vi "DDS_Check_Box.vi"(8 "error in (no error)":errorcluster, 10 "box #":i32, 11 "DDS Settings":T1={"Enable DDS"=TRUE, "Array of DDS Boxes"=[{"DDS box device reference"={"NI USB-8451 device reference"="USB0::0x3923::0x7166::01574F57::RAW", "DIO port"=0, "Serial Clock Rate [kHz]"=1000}, "Array of DDS Channels (4)"=[{"Power"=TRUE, "Channel Parameters"={"Ref Clock Rate [kHz]"=1000.0, "Full Scale Output\nPower [dBm]"=0.0}, "RAM Enable"=FALSE, "RAM Dest Type"=0, "RAM Default"={"Frequency [MHz]"="20", "Amplitude [dBm]"="-15", "Phase Offset [rad]"="0"}, "Array of DDS Profiles (8)"=[{"Single Tone"={"Frequency [MHz]"="75", "Amplitude [dBm]"="0", "Phase Offset [rad]"="0"}, "RAM Mode "=enum."Ramp Up", "Zero-crossing"=FALSE, "No Dwell High"=FALSE, "Function/Static"=TRUE, "RAM Function Settings"=["10*x", "1", "1", "260", "10"], "RAM Static Array"=[0.0], "Description"=""}, {"Single Tone"={"Frequency [MHz]"="200", "Amplitude [dBm]"="0", "Phase Offset [rad]"="0"}, "RAM Mode "=enum."Direct Switch", "Zero-crossing"=FALSE, "No Dwell High"=FALSE, "Function/Static"=FALSE, "RAM Function Settings"=["", "", "", "", "1"], "RAM Static Array"=[0.0], "Description"=""}, {"Single Tone"={"Frequency [MHz]"="", "Amplitude [dBm]"="", "Phase Offset [rad]"="0"}, "RAM Mode "=enum."Direct Switch", "Zero-crossing"=FALSE, "No Dwell High"=FALSE, "Function/Static"=FALSE, "RAM Function Settings"=["", "", "", "", "1"], "RAM Static Array"=[0.0], "Description"=""}, {"Single Tone"={"Frequency [MHz]"="", "Amplitude [dBm]"="0", "Phase Offset [rad]"="0"}, "RAM Mode "=enum."Ramp Up", "Zero-crossing"=FALSE, "No Dwell High"=FALSE, "Function/Static"=FALSE, "RAM Function Settings"=["10*x", "1", "1", "260", "10"], "RAM Static Array"=[0.0], "Description"=""}, {"Single Tone"={"Frequency [MHz]"="0", "Amplitude [dBm]"="-50", "Phase Offset [rad]"="0"}, "RAM Mode "=enum."Direct Switch", "Zero-crossing"=FALSE, "No Dwell High"=FALSE, "Function/Static"=FALSE, "RAM Function Settings"=["", "", "", "", "1"], "RAM Static Array"=[0.0], "Description"=""}, {"Single Tone"={"Frequency [MHz]"="0", "Amplitude [dBm]"="-50", "Phase Offset [rad]"="0"}, "RAM Mode "=enum."Direct Switch", "Zero-crossing"=FALSE, "No Dwell High"=FALSE, "Function/Static"=FALSE, "RAM Function Settings"=["", "", "", "", "1"], "RAM Static Array"=[0.0], "Description"=""}, {"Single Tone"={"Frequency [MHz]"="0", "Amplitude [dBm]"="-50", "Phase Offset [rad]"="0"}, "RAM Mode "=enum."Direct Switch", "Zero-crossing"=FALSE, "No Dwell High"=FALSE, "Function/Static"=FALSE, "RAM Function Settings"=["", "", "", "", "1"], "RAM Static Array"=[0.0], "Description"=""}, {"Single Tone"={"Frequency [MHz]"="0", "Amplitude [dBm]"="-50", "Phase Offset [rad]"="0"}, "RAM Mode "=enum."Direct Switch", "Zero-crossing"=FALSE, "No Dwell High"=FALSE, "Function/Static"=FALSE, "RAM Function Settings"=["", "", "", "", "1"], "RAM Static Array"=[0.0], "Description"=""}], "Description"=""}, {"Power"=TRUE, "Channel Parameters"={"Ref Clock Rate [kHz]"=1000.0, "Full Scale Output\nPower [dBm]"=0.0}, "RAM Enable"=FALSE, "RAM Dest Type"=0, "RAM Default"={"Frequency [MHz]"="", "Amplitude [dBm]"="-50", "Phase Offset [rad]"=""}, "Array of DDS Profiles (8)"=[{"Single Tone"={"Frequency [MHz]"="278.5", "Amplitude [dBm]"="0", "Phase Offset [rad]"="0"}, "RAM Mode "=enum."Direct Switch", "Zero-crossing"=FALSE, "No Dwell High"=FALSE, "Function/Static"=TRUE, "RAM Function Settings"=["", "", "", "", "1"], "RAM Static Array"=[0.0], "Description"=""}, {"Single Tone"={"Frequency [MHz]"="278.5", "Amplitude [dBm]"="-150", "Phase Offset [rad]"="0"}, "RAM Mode "=enum."Direct Switch", "Zero-crossing"=FALSE, "No Dwell High"=FALSE, "Function/Static"=FALSE, "RAM Function Settings"=["", "", "", "", "1"], "RAM Static Array"=[0.0], "Description"=""}, {"Single Tone"={"Frequency [MHz]"="278.5", "Amplitude [dBm]"="-10", "Phase Offset [rad]"="0"}, "RAM Mode "=enum."Direct Switch", "Zero-crossing"=FALSE, "No Dwell High"=FALSE, "Function/Static"=FALSE, "RAM Function Settings"=["", "", "", "", "1"], "RAM Static Array"=[0.0], "Description"=""}, {"Single Tone"={"Frequency [MHz]"="278.5", "Amplitude [dBm]"="-10", "Phase Offset [rad]"="0"}, "RAM Mode "=enum."Direct Switch", "Zero-crossing"=FALSE, "No Dwell High"=FALSE, "Function/Static"=FALSE, "RAM Function Settings"=["", "", "", "", "1"], "RAM Static Array"=[0.0], "Description"=""}, {"Single Tone"={"Frequency [MHz]"="60", "Amplitude [dBm]"="-50", "Phase Offset [rad]"="0"}, "RAM Mode "=enum."Direct Switch", "Zero-crossing"=FALSE, "No Dwell High"=FALSE, "Function/Static"=FALSE, "RAM Function Settings"=["", "", "", "", "1"], "RAM Static Array"=[0.0], "Description"=""}, {"Single Tone"={"Frequency [MHz]"="70", "Amplitude [dBm]"="-50", "Phase Offset [rad]"="0"}, "RAM Mode "=enum."Direct Switch", "Zero-crossing"=FALSE, "No Dwell High"=FALSE, "Function/Static"=FALSE, "RAM Function Settings"=["", "", "", "", "1"], "RAM Static Array"=[0.0], "Description"=""}, {"Single Tone"={"Frequency [MHz]"="80", "Amplitude [dBm]"="-50", "Phase Offset [rad]"="0"}, "RAM Mode "=enum."Direct Switch", "Zero-crossing"=FALSE, "No Dwell High"=FALSE, "Function/Static"=FALSE, "RAM Function Settings"=["", "", "", "", "1"], "RAM Static Array"=[0.0], "Description"=""}, {"Single Tone"={"Frequency [MHz]"="90", "Amplitude [dBm]"="-50", "Phase Offset [rad]"="0"}, "RAM Mode "=enum."Direct Switch", "Zero-crossing"=FALSE, "No Dwell High"=FALSE, "Function/Static"=FALSE, "RAM Function Settings"=["", "", "", "", "1"], "RAM Static Array"=[0.0], "Description"=""}], "Description"=""}, {"Power"=TRUE, "Channel Parameters"={"Ref Clock Rate [kHz]"=1000.0, "Full Scale Output\nPower [dBm]"=0.0}, "RAM Enable"=FALSE, "RAM Dest Type"=0, "RAM Default"={"Frequency [MHz]"="", "Amplitude [dBm]"="-50", "Phase Offset [rad]"=""}, "Array of DDS Profiles (8)"=[{"Single Tone"={"Frequency [MHz]"="108", "Amplitude [dBm]"="0", "Phase Offset [rad]"="0"}, "RAM Mode "=enum."Direct Switch", "Zero-crossing"=FALSE, "No Dwell High"=FALSE, "Function/Static"=TRUE, "RAM Function Settings"=["", "", "", "", "1"], "RAM Static Array"=[0.0], "Description"=""}, {"Single Tone"={"Frequency [MHz]"="93", "Amplitude [dBm]"="-4", "Phase Offset [rad]"="0"}, "RAM Mode "=enum."Direct Switch", "Zero-crossing"=FALSE, "No Dwell High"=FALSE, "Function/Static"=FALSE, "RAM Function Settings"=["", "", "", "", "1"], "RAM Static Array"=[0.0], "Description"=""}, {"Single Tone"={"Frequency [MHz]"="95", "Amplitude [dBm]"="-150", "Phase Offset [rad]"="0"}, "RAM Mode "=enum."Direct Switch", "Zero-crossing"=FALSE, "No Dwell High"=FALSE, "Function/Static"=FALSE, "RAM Function Settings"=["", "", "", "", "1"], "RAM Static Array"=[0.0], "Description"=""}, {"Single Tone"={"Frequency [MHz]"="96", "Amplitude [dBm]"="-3", "Phase Offset [rad]"="0"}, "RAM Mode "=enum."Direct Switch", "Zero-crossing"=FALSE, "No Dwell High"=FALSE, "Function/Static"=FALSE, "RAM Function Settings"=["", "", "", "", "1"], "RAM Static Array"=[0.0], "Description"=""}, {"Single Tone"={"Frequency [MHz]"="0", "Amplitude [dBm]"="-50", "Phase Offset [rad]"="0"}, "RAM Mode "=enum."Direct Switch", "Zero-crossing"=FALSE, "No Dwell High"=FALSE, "Function/Static"=FALSE, "RAM Function Settings"=["", "", "", "", "1"], "RAM Static Array"=[0.0], "Description"=""}, {"Single Tone"={"Frequency [MHz]"="0", "Amplitude [dBm]"="-50", "Phase Offset [rad]"="0"}, "RAM Mode "=enum."Direct Switch", "Zero-crossing"=FALSE, "No Dwell High"=FALSE, "Function/Static"=FALSE, "RAM Function Settings"=["", "", "", "", "1"], "RAM Static Array"=[0.0], "Description"=""}, {"Single Tone"={"Frequency [MHz]"="0", "Amplitude [dBm]"="-50", "Phase Offset [rad]"="0"}, "RAM Mode "=enum."Direct Switch", "Zero-crossing"=FALSE, "No Dwell High"=FALSE, "Function/Static"=FALSE, "RAM Function Settings"=["", "", "", "", "1"], "RAM Static Array"=[0.0], "Description"=""}, {"Single Tone"={"Frequency [MHz]"="0", "Amplitude [dBm]"="-50", "Phase Offset [rad]"="0"}, "RAM Mode "=enum."Direct Switch", "Zero-crossing"=FALSE, "No Dwell High"=FALSE, "Function/Static"=FALSE, "RAM Function Settings"=["", "", "", "", "1"], "RAM Static Array"=[0.0], "Description"=""}], "Description"=""}, {"Power"=TRUE, "Channel Parameters"={"Ref Clock Rate [kHz]"=1000.0, "Full Scale Output\nPower [dBm]"=0.0}, "RAM Enable"=FALSE, "RAM Dest Type"=0, "RAM Default"={"Frequency [MHz]"="", "Amplitude [dBm]"="-50", "Phase Offset [rad]"=""}, "Array of DDS Profiles (8)"=[{"Single Tone"={"Frequency [MHz]"="y", "Amplitude [dBm]"="0", "Phase Offset [rad]"="0"}, "RAM Mode "=enum."Direct Switch", "Zero-crossing"=FALSE, "No Dwell High"=FALSE, "Function/Static"=TRUE, "RAM Function Settings"=["", "", "", "", "1"], "RAM Static Array"=[0.0], "Description"=""}, {"Single Tone"={"Frequency [MHz]"="75", "Amplitude [dBm]"="0", "Phase Offset [rad]"="0"}, "RAM Mode "=enum."Direct Switch", "Zero-crossing"=FALSE, "No Dwell High"=FALSE, "Function/Static"=FALSE, "RAM Function Settings"=["", "", "", "", "1"], "RAM Static Array"=[0.0], "Description"=""}, {"Single Tone"={"Frequency [MHz]"="0", "Amplitude [dBm]"="-50", "Phase Offset [rad]"="0"}, "RAM Mode "=enum."Direct Switch", "Zero-crossing"=FALSE, "No Dwell High"=FALSE, "Function/Static"=FALSE, "RAM Function Settings"=["", "", "", "", "1"], "RAM Static Array"=[0.0], "Description"=""}, {"Single Tone"={"Frequency [MHz]"="0", "Amplitude [dBm]"="-50", "Phase Offset [rad]"="0"}, "RAM Mode "=enum."Direct Switch", "Zero-crossing"=FALSE, "No Dwell High"=FALSE, "Function/Static"=FALSE, "RAM Function Settings"=["", "", "", "", "1"], "RAM Static Array"=[0.0], "Description"=""}, {"Single Tone"={"Frequency [MHz]"="0", "Amplitude [dBm]"="-50", "Phase Offset [rad]"="0"}, "RAM Mode "=enum."Direct Switch", "Zero-crossing"=FALSE, "No Dwell High"=FALSE, "Function/Static"=FALSE, "RAM Function Settings"=["", "", "", "", "1"], "RAM Static Array"=[0.0], "Description"=""}, {"Single Tone"={"Frequency [MHz]"="0", "Amplitude [dBm]"="-50", "Phase Offset [rad]"="0"}, "RAM Mode "=enum."Direct Switch", "Zero-crossing"=FALSE, "No Dwell High"=FALSE, "Function/Static"=FALSE, "RAM Function Settings"=["", "", "", "", "1"], "RAM Static Array"=[0.0], "Description"=""}, {"Single Tone"={"Frequency [MHz]"="0", "Amplitude [dBm]"="-50", "Phase Offset [rad]"="0"}, "RAM Mode "=enum."Direct Switch", "Zero-crossing"=FALSE, "No Dwell High"=FALSE, "Function/Static"=FALSE, "RAM Function Settings"=["", "", "", "", "1"], "RAM Static Array"=[0.0], "Description"=""}, {"Single Tone"={"Frequency [MHz]"="0", "Amplitude [dBm]"="-50", "Phase Offset [rad]"="0"}, "RAM Mode "=enum."Direct Switch", "Zero-crossing"=FALSE, "No Dwell High"=FALSE, "Function/Static"=FALSE, "RAM Function Settings"=["", "", "", "", "1"], "RAM Static Array"=[0.0], "Description"=""}], "Description"=""}], "Enable"=TRUE, "Description"=""}, {"DDS box device reference"={"NI USB-8451 device reference"="USB0::0x3923::0x7166::01574FA5::RAW", "DIO port"=0, "Serial Clock Rate [kHz]"=1000}, "Array of DDS Channels (4)"=[{"Power"=TRUE, "Channel Parameters"={"Ref Clock Rate [kHz]"=1000.0, "Full Scale Output\nPower [dBm]"=0.0}, "RAM Enable"=FALSE, "RAM Dest Type"=2, "RAM Default"={"Frequency [MHz]"="150", "Amplitude [dBm]"="0", "Phase Offset [rad]"="0"}, "Array of DDS Profiles (8)"=[{"Single Tone"={"Frequency [MHz]"="150", "Amplitude [dBm]"="0", "Phase Offset [rad]"="0"}, "RAM Mode "=enum."Direct Switch", "Zero-crossing"=FALSE, "No Dwell High"=FALSE, "Function/Static"=FALSE, "RAM Function Settings"=[], "RAM Static Array"=[0.0, -0.0477, -0.173, -0.327, -0.452, -0.5], "Description"=""}, {"Single Tone"={"Frequency [MHz]"="150", "Amplitude [dBm]"="-.5", "Phase Offset [rad]"="0"}, "RAM Mode "=enum."Continuous Recirculate", "Zero-crossing"=FALSE, "No Dwell High"=FALSE, "Function/Static"=FALSE, "RAM Function Settings"=["", "", "", "1000000/f/10", "10"], "RAM Static Array"=[0.0, -1.0, -2.0, -3.0, -4.0], "Description"=""}, {"Single Tone"={"Frequency [MHz]"="150", "Amplitude [dBm]"="0", "Phase Offset [rad]"="0"}, "RAM Mode "=enum."Direct Switch", "Zero-crossing"=FALSE, "No Dwell High"=FALSE, "Function/Static"=FALSE, "RAM Function Settings"=[], "RAM Static Array"=[0.0, 0.0, 0.0, 0.0, 0.0, 0.0], "Description"=""}, {"Single Tone"={"Frequency [MHz]"="150", "Amplitude [dBm]"="0", "Phase Offset [rad]"="0"}, "RAM Mode "=enum."Direct Switch", "Zero-crossing"=FALSE, "No Dwell High"=FALSE, "Function/Static"=FALSE, "RAM Function Settings"=[], "RAM Static Array"=[0.0, 0.0, 0.0, 0.0, 0.0, 0.0], "Description"=""}, {"Single Tone"={"Frequency [MHz]"="157.5", "Amplitude [dBm]"="0", "Phase Offset [rad]"="0"}, "RAM Mode "=enum."Direct Switch", "Zero-crossing"=FALSE, "No Dwell High"=FALSE, "Function/Static"=FALSE, "RAM Function Settings"=[], "RAM Static Array"=[], "Description"=""}, {"Single Tone"={"Frequency [MHz]"="157.5", "Amplitude [dBm]"="0", "Phase Offset [rad]"="0"}, "RAM Mode "=enum."Direct Switch", "Zero-crossing"=FALSE, "No Dwell High"=FALSE, "Function/Static"=FALSE, "RAM Function Settings"=[], "RAM Static Array"=[], "Description"=""}, {"Single Tone"={"Frequency [MHz]"="157.5", "Amplitude [dBm]"="0", "Phase Offset [rad]"="0"}, "RAM Mode "=enum."Direct Switch", "Zero-crossing"=FALSE, "No Dwell High"=FALSE, "Function/Static"=FALSE, "RAM Function Settings"=[], "RAM Static Array"=[], "Description"=""}, {"Single Tone"={"Frequency [MHz]"="157.5", "Amplitude [dBm]"="0", "Phase Offset [rad]"="0"}, "RAM Mode "=enum."Direct Switch", "Zero-crossing"=FALSE, "No Dwell High"=FALSE, "Function/Static"=FALSE, "RAM Function Settings"=[], "RAM Static Array"=[], "Description"=""}], "Description"=""}, {"Power"=TRUE, "Channel Parameters"={"Ref Clock Rate [kHz]"=1000.0, "Full Scale Output\nPower [dBm]"=0.0}, "RAM Enable"=FALSE, "RAM Dest Type"=0, "RAM Default"={"Frequency [MHz]"="", "Amplitude [dBm]"="", "Phase Offset [rad]"=""}, "Array of DDS Profiles (8)"=[{"Single Tone"={"Frequency [MHz]"="150", "Amplitude [dBm]"="0", "Phase Offset [rad]"="0"}, "RAM Mode "=enum."Direct Switch", "Zero-crossing"=FALSE, "No Dwell High"=FALSE, "Function/Static"=FALSE, "RAM Function Settings"=["", "", "", "1000000/f/10", "10"], "RAM Static Array"=[0.0, -1.0, -2.0, -3.0, -4.0, 0.0], "Description"=""}, {"Single Tone"={"Frequency [MHz]"="150", "Amplitude [dBm]"="-150", "Phase Offset [rad]"="0"}, "RAM Mode "=enum."Direct Switch", "Zero-crossing"=FALSE, "No Dwell High"=FALSE, "Function/Static"=FALSE, "RAM Function Settings"=[], "RAM Static Array"=[0.0, 0.0, 0.0, 0.0, 0.0], "Description"=""}, {"Single Tone"={"Frequency [MHz]"="150", "Amplitude [dBm]"="0", "Phase Offset [rad]"="0"}, "RAM Mode "=enum."Direct Switch", "Zero-crossing"=FALSE, "No Dwell High"=FALSE, "Function/Static"=FALSE, "RAM Function Settings"=[], "RAM Static Array"=[0.0, 0.0, 0.0, 0.0, 0.0, 0.0], "Description"=""}, {"Single Tone"={"Frequency [MHz]"="150", "Amplitude [dBm]"="0", "Phase Offset [rad]"="0"}, "RAM Mode "=enum."Direct Switch", "Zero-crossing"=FALSE, "No Dwell High"=FALSE, "Function/Static"=FALSE, "RAM Function Settings"=[], "RAM Static Array"=[], "Description"=""}, {"Single Tone"={"Frequency [MHz]"="157.5", "Amplitude [dBm]"="0", "Phase Offset [rad]"="0"}, "RAM Mode "=enum."Direct Switch", "Zero-crossing"=FALSE, "No Dwell High"=FALSE, "Function/Static"=FALSE, "RAM Function Settings"=[], "RAM Static Array"=[], "Description"=""}, {"Single Tone"={"Frequency [MHz]"="157.5", "Amplitude [dBm]"="0", "Phase Offset [rad]"="0"}, "RAM Mode "=enum."Direct Switch", "Zero-crossing"=FALSE, "No Dwell High"=FALSE, "Function/Static"=FALSE, "RAM Function Settings"=[], "RAM Static Array"=[], "Description"=""}, {"Single Tone"={"Frequency [MHz]"="157.5", "Amplitude [dBm]"="-22", "Phase Offset [rad]"="0"}, "RAM Mode "=enum."Direct Switch", "Zero-crossing"=FALSE, "No Dwell High"=FALSE, "Function/Static"=FALSE, "RAM Function Settings"=[], "RAM Static Array"=[], "Description"=""}, {"Single Tone"={"Frequency [MHz]"="157.5", "Amplitude [dBm]"="-22", "Phase Offset [rad]"="0"}, "RAM Mode "=enum."Direct Switch", "Zero-crossing"=FALSE, "No Dwell High"=FALSE, "Function/Static"=FALSE, "RAM Function Settings"=[], "RAM Static Array"=[], "Description"=""}], "Description"=""}, {"Power"=TRUE, "Channel Parameters"={"Ref Clock Rate [kHz]"=1000.0, "Full Scale Output\nPower [dBm]"=0.0}, "RAM Enable"=FALSE, "RAM Dest Type"=0, "RAM Default"={"Frequency [MHz]"="", "Amplitude [dBm]"="", "Phase Offset [rad]"=""}, "Array of DDS Profiles (8)"=[{"Single Tone"={"Frequency [MHz]"="150", "Amplitude [dBm]"="0", "Phase Offset [rad]"="0"}, "RAM Mode "=enum."Direct Switch", "Zero-crossing"=FALSE, "No Dwell High"=FALSE, "Function/Static"=FALSE, "RAM Function Settings"=[], "RAM Static Array"=[0.0, 0.0, 0.0, 0.0, 0.0, 0.0], "Description"=""}, {"Single Tone"={"Frequency [MHz]"="150", "Amplitude [dBm]"="0", "Phase Offset [rad]"="0"}, "RAM Mode "=enum."Direct Switch", "Zero-crossing"=FALSE, "No Dwell High"=FALSE, "Function/Static"=FALSE, "RAM Function Settings"=[], "RAM Static Array"=[0.0, 0.0, 0.0, 0.0, 0.0], "Description"=""}, {"Single Tone"={"Frequency [MHz]"="157.5", "Amplitude [dBm]"="-22", "Phase Offset [rad]"="0"}, "RAM Mode "=enum."Direct Switch", "Zero-crossing"=FALSE, "No Dwell High"=FALSE, "Function/Static"=FALSE, "RAM Function Settings"=[], "RAM Static Array"=[], "Description"=""}, {"Single Tone"={"Frequency [MHz]"="157.5", "Amplitude [dBm]"="-22", "Phase Offset [rad]"="0"}, "RAM Mode "=enum."Direct Switch", "Zero-crossing"=FALSE, "No Dwell High"=FALSE, "Function/Static"=FALSE, "RAM Function Settings"=[], "RAM Static Array"=[], "Description"=""}, {"Single Tone"={"Frequency [MHz]"="157.5", "Amplitude [dBm]"="-22", "Phase Offset [rad]"="0"}, "RAM Mode "=enum."Direct Switch", "Zero-crossing"=FALSE, "No Dwell High"=FALSE, "Function/Static"=FALSE, "RAM Function Settings"=[], "RAM Static Array"=[], "Description"=""}, {"Single Tone"={"Frequency [MHz]"="157.5", "Amplitude [dBm]"="-22", "Phase Offset [rad]"="0"}, "RAM Mode "=enum."Direct Switch", "Zero-crossing"=FALSE, "No Dwell High"=FALSE, "Function/Static"=FALSE, "RAM Function Settings"=[], "RAM Static Array"=[], "Description"=""}, {"Single Tone"={"Frequency [MHz]"="157.5", "Amplitude [dBm]"="-22", "Phase Offset [rad]"="0"}, "RAM Mode "=enum."Direct Switch", "Zero-crossing"=FALSE, "No Dwell High"=FALSE, "Function/Static"=FALSE, "RAM Function Settings"=[], "RAM Static Array"=[], "Description"=""}, {"Single Tone"={"Frequency [MHz]"="150", "Amplitude [dBm]"="0", "Phase Offset [rad]"="0"}, "RAM Mode "=enum."Direct Switch", "Zero-crossing"=FALSE, "No Dwell High"=FALSE, "Function/Static"=FALSE, "RAM Function Settings"=[], "RAM Static Array"=[], "Description"=""}], "Description"=""}, {"Power"=TRUE, "Channel Parameters"={"Ref Clock Rate [kHz]"=1000.0, "Full Scale Output\nPower [dBm]"=0.0}, "RAM Enable"=FALSE, "RAM Dest Type"=0, "RAM Default"={"Frequency [MHz]"="", "Amplitude [dBm]"="", "Phase Offset [rad]"=""}, "Array of DDS Profiles (8)"=[{"Single Tone"={"Frequency [MHz]"="165", "Amplitude [dBm]"="0", "Phase Offset [rad]"="0"}, "RAM Mode "=enum."Direct Switch", "Zero-crossing"=FALSE, "No Dwell High"=FALSE, "Function/Static"=FALSE, "RAM Function Settings"=[], "RAM Static Array"=[0.0, 0.0, 0.0, 0.0, 0.0, 0.0], "Description"=""}, {"Single Tone"={"Frequency [MHz]"="165", "Amplitude [dBm]"="0", "Phase Offset [rad]"="0"}, "RAM Mode "=enum."Direct Switch", "Zero-crossing"=FALSE, "No Dwell High"=FALSE, "Function/Static"=FALSE, "RAM Function Settings"=[], "RAM Static Array"=[], "Description"=""}, {"Single Tone"={"Frequency [MHz]"="157.5", "Amplitude [dBm]"="-22", "Phase Offset [rad]"="0"}, "RAM Mode "=enum."Direct Switch", "Zero-crossing"=FALSE, "No Dwell High"=FALSE, "Function/Static"=FALSE, "RAM Function Settings"=[], "RAM Static Array"=[], "Description"=""}, {"Single Tone"={"Frequency [MHz]"="157.5", "Amplitude [dBm]"="-22", "Phase Offset [rad]"="0"}, "RAM Mode "=enum."Direct Switch", "Zero-crossing"=FALSE, "No Dwell High"=FALSE, "Function/Static"=FALSE, "RAM Function Settings"=[], "RAM Static Array"=[], "Description"=""}, {"Single Tone"={"Frequency [MHz]"="157.5", "Amplitude [dBm]"="-22", "Phase Offset [rad]"="0"}, "RAM Mode "=enum."Direct Switch", "Zero-crossing"=FALSE, "No Dwell High"=FALSE, "Function/Static"=FALSE, "RAM Function Settings"=[], "RAM Static Array"=[], "Description"=""}, {"Single Tone"={"Frequency [MHz]"="157.5", "Amplitude [dBm]"="-22", "Phase Offset [rad]"="0"}, "RAM Mode "=enum."Direct Switch", "Zero-crossing"=FALSE, "No Dwell High"=FALSE, "Function/Static"=FALSE, "RAM Function Settings"=[], "RAM Static Array"=[], "Description"=""}, {"Single Tone"={"Frequency [MHz]"="157.5", "Amplitude [dBm]"="-22", "Phase Offset [rad]"="0"}, "RAM Mode "=enum."Direct Switch", "Zero-crossing"=FALSE, "No Dwell High"=FALSE, "Function/Static"=FALSE, "RAM Function Settings"=[], "RAM Static Array"=[], "Description"=""}, {"Single Tone"={"Frequency [MHz]"="150", "Amplitude [dBm]"="0", "Phase Offset [rad]"="0"}, "RAM Mode "=enum."Direct Switch", "Zero-crossing"=FALSE, "No Dwell High"=FALSE, "Function/Static"=FALSE, "RAM Function Settings"=[], "RAM Static Array"=[], "Description"=""}], "Description"=""}], "Enable"=TRUE, "Description"=""}]} {"Array of DDS Boxes"."Array of DDS Channels (4)"."Channel Parameters"."Ref Clock Rate [kHz]" min=0.0}) -> (0 "error out":errorcluster, 1 "CFR3":u8[][](array[numeric]), 2 "CFR2":u8[][](array[numeric]), 3 "CFR1":u8[][](array[numeric]))   [LabVIEW 2013]
uses:
  cesium_controller/DDS/DDS_Settings_Cluster.ctl
  Array_of_DDS_Boxes.ctl
  DDS_box_cluster.ctl
  DDS_box_device_reference.ctl
  <vilib>/ni845x/ni845x.llb/ni845xControl.ctl
  array_of_DDS_channels.ctl
  DDS_channel.ctl
  array_of_DDS_profiles.ctl
  DDS_profile.ctl
  DDS RAM mode.ctl
  AD9910 registers.ctl
  cesium_controller/DDS/DDS.lvclass
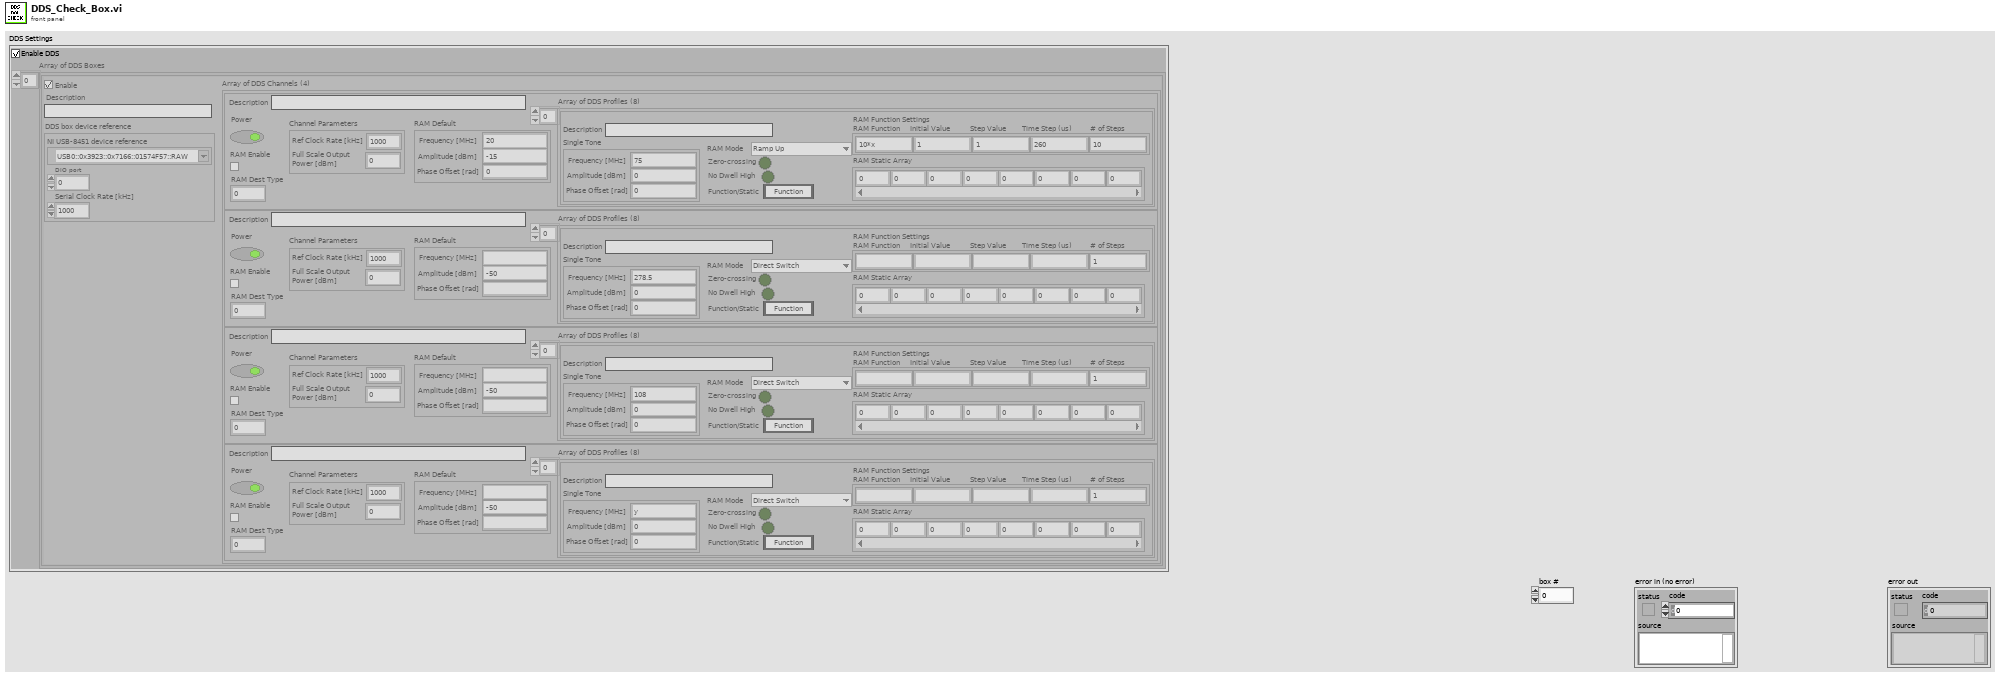
[diagram p1: front panel]
types:
  T1 = typedef "DDS_Settings_Cluster.ctl" = cluster{"Enable DDS":bool, "Array of DDS Boxes":T2}
  T2 = typedef "Array_of_DDS_Boxes.ctl" = T3[]
  T3 = typedef "DDS_box_cluster.ctl" = cluster{"DDS box device reference":T4, "Array of DDS Channels (4)":T6, "Enable":bool, "Description":string}
  T4 = typedef "DDS_box_device_reference.ctl" = cluster{"NI USB-8451 device reference":T5, "DIO port":u8, "Serial Clock Rate [kHz]":u16}
  T5 = typedef "ni845xControl.ctl" = refnum<k21>
  T6 = typedef "DDS.lvclass/array_of_DDS_channels.ctl" = T7[]
  T7 = typedef "DDS.lvclass/DDS_channel.ctl" = cluster{"Power":bool, "Channel Parameters":cluster{"Ref Clock Rate [kHz]":dbl, "Full Scale Output\nPower [dBm]":dbl}, "RAM Enable":bool, "RAM Dest Type":u8, "RAM Default":cluster{"Frequency [MHz]":string, "Amplitude [dBm]":string, "Phase Offset [rad]":string}, "Array of DDS Profiles (8)":T8, "Description":string}
  T8 = typedef "DDS.lvclass/array_of_DDS_profiles.ctl" = T9[]
  T9 = typedef "DDS_profile.ctl" = cluster{"Single Tone":cluster{"Frequency [MHz]":string, "Amplitude [dBm]":string, "Phase Offset [rad]":string}, "RAM Mode ":T10, "Zero-crossing":bool, "No Dwell High":bool, "Function/Static":bool, "RAM Function Settings":string[], "RAM Static Array":dbl[], "Description":string}
  T10 = typedef "DDS RAM mode.ctl" = enum16{"Direct Switch", "Ramp Up", "Bidirectional Ramp", "Continuous Bidirectional Ramp", "Continuous Recirculate", "Direct Switch 2", "Direct Switch 3", "Direct Switch 4"}
  T11 = typedef "AD9910 registers.ctl" = enum16{"CFR1", "CFR2", "CFR3", "Auxiliary DAC Control", "I/0 Update Rate", "Frequency Tuning Word", "Phase Offset Word", "Amplitude Scale Factor", "Multichip Sync", "Digital Ramp Limit", "Digital Ramp Step Size", "Digital Ramp Rate", "Single Tone Profile 0", "Single Tone Profile 1", "Single Tone Profile 2", "Single Tone Profile 3", "Single Tone Profile 4", "Single Tone Profile 5", "Single Tone Profile 6", "Single Tone Profile 7", "RAM Profile 0", "RAM Profile 1", "RAM Profile 2", "RAM Profile 3", "RAM Profile 4", "RAM Profile 5", "RAM Profile 6", "RAM Profile 7", "RAM"}
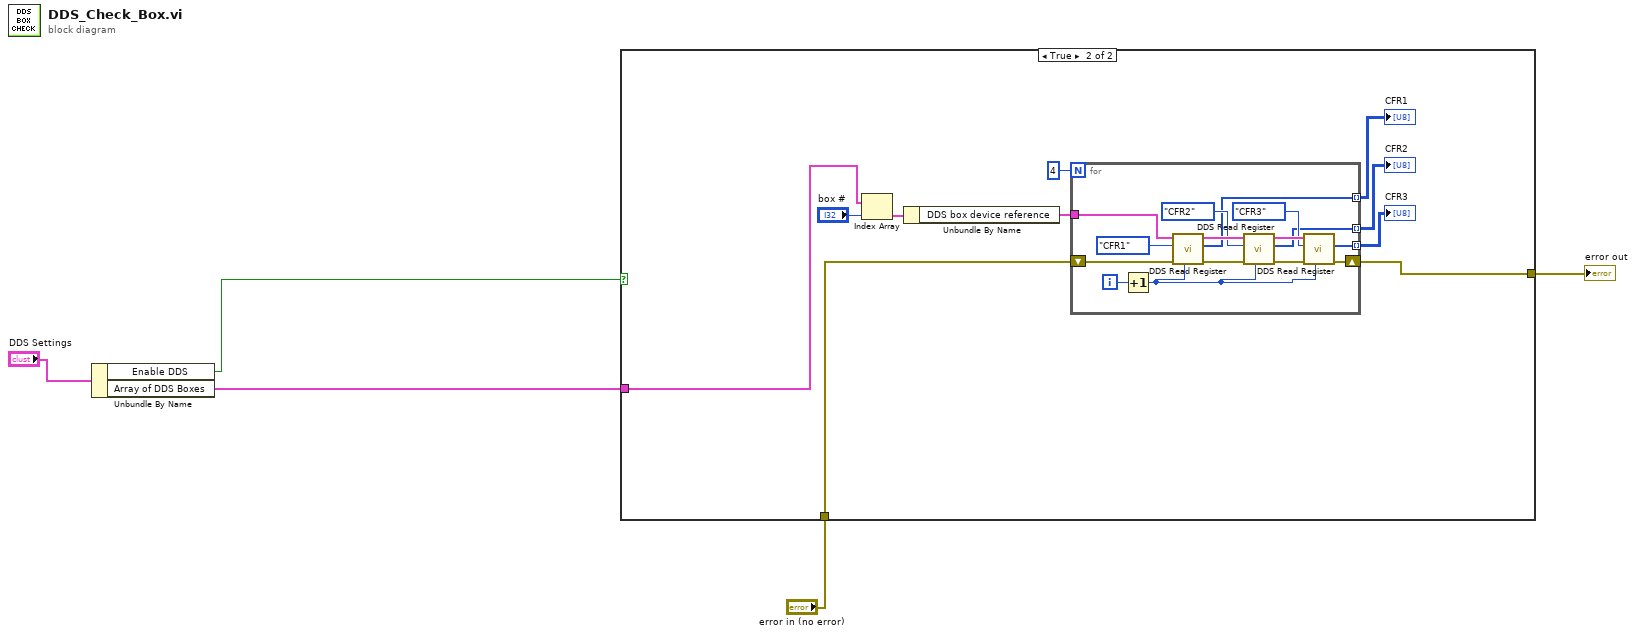
[diagram p0: block diagram]
diagram:
  n1 = Unbundle By Name("DDS Settings") -> ("Enable DDS"=w3:bool, "Array of DDS Boxes"=w4:T2)
  n2 = case shown="True" w3 {
    tunnel: w4 -> [_ w9]
    tunnel: "error in (no error)" -> [w6 w8]
    tunnel: [w6 w7] -> w1
    frame False {
    }
    frame True {
      n3 = Index Array(array=w9, index="box #") -> (element=w12:T3)
      n4 = Unbundle By Name(w12) -> ("DDS box device reference"=w11:T4)
      n5 = for {
        N: 4 -> [_]
        tunnel: w11 -> [w31]
        tunnel: [w20] -> w15 mode=indexing
        tunnel: [w19] -> w14 mode=indexing
        tunnel: [w18] -> w13 mode=indexing
        shift-right: [w17] -> w7
        shift-left: w8 -> [w30]
        i -> [w29]
        n6 = Increment(x=w29) -> (x+1=w21:i32)
        n7 = call "DDS Read Register.vi"("channel number (1)"=w21, "error in (no error)"=w30, "Register"=AD9910_registers."CFR1", "DDS ref in"=w31) -> ("error out"=w26:errorcluster, "Read data"=w20:u8[], "DDS ref out"=w27:T4)  [unwired: 5 in]
        n8 = call "DDS Read Register.vi"("channel number (1)"=w21, "error in (no error)"=w26, "Register"=AD9910_registers."CFR2", "DDS ref in"=w27) -> ("error out"=w25:errorcluster, "Read data"=w19:u8[], "DDS ref out"=w24:T4)  [unwired: 5 in]
        n9 = call "DDS Read Register.vi"("channel number (1)"=w21, "error in (no error)"=w25, "Register"=AD9910_registers."CFR3", "DDS ref in"=w24) -> ("error out"=w17:errorcluster, "Read data"=w18:u8[])  [unwired: 5 in, 1 out]
      }
      "CFR1" <- w15
      "CFR2" <- w14
      "CFR3" <- w13
    }
  }
  "error out" <- w1
